vi "PNDT - test number to scan index.vi"(4 "reset":bool, 5 "test no.":i32) -> (1 "#scans":i32, 2 "scan index":i32)   [LabVIEW 2026, in "MicroPulse_Driver.lvlib"]
doc: "Normalise PA test numbers to zero based index"
uses:
  MicroPulse_Driver.lvlib
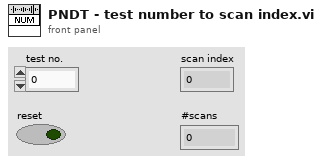
[diagram p1: front panel]
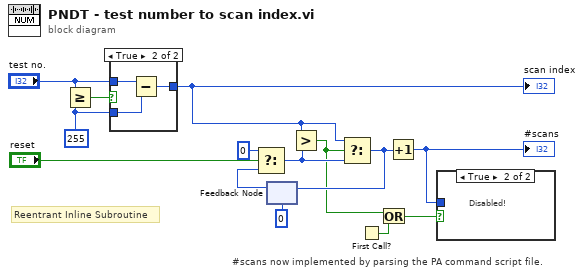
[diagram p0: block diagram]
diagram:
  w13 = 255 ("y")
  # "#scans now implemented by parsing the PA command script file."
  # "Reentrant Inline Subroutine"
  n1 = Greater Or Equal?(x="test no.", y=w13) -> (x >= y?=w12:bool)
  n2 = case shown="True" w12 {
    tunnel: [w15 w18] -> w11
    tunnel: "test no." -> [w15 w17]
    tunnel: w13 -> [_ w16]
    frame False {
    }
    frame True {
      n3 = Subtract(x=w17, y=w16) -> (x-y=w18:i32)
    }
  }
  "scan index" <- w11
  n4 = feedback #1(0 ("t")) -> (w8:i32)
  n5 = Select(t=0, s="reset", f=w8) -> (s? t:f=w7:i32)
  n6 = Greater?(x=w11, y=w7) -> (0:w2:bool)
  n7 = Select(t=w11, s=w2, f=w7) -> (s? t:f=w9:i32)
  n8 = feedback-in #1(w9) -> ()
  n9 = First Call?() -> (First Call?: T/F=w3:bool)
  n10 = Or(x=w2, y=w3) -> (x .or. y?=w1:bool)
  n11 = Increment(x=w9) -> (x+1=w4:i32)
  "#scans" <- w4
  n12 = case shown="True" w1 {
    tunnel: w4 -> [_ _]
    frame False {
    }
    frame True {
      # "Disabled!"
    }
  }
